vi "Get latest RSS.vi"(8 "error in (no error)":errorcluster, 10 "software sets":T1[](array[typedef]) {"information"."component type" items=["standard", "hidden", "system", "unknown", "startup"]; "items"."component type" items=["standard", "hidden", "system", "unknown", "startup"]; "add-ons"."component type" items=["standard", "hidden", "system", "unknown", "startup"]}) -> (0 "error out":errorcluster, 2 "software set":T1 {"information"."component type" items=["standard", "hidden", "system", "unknown", "startup"]; "items"."component type" items=["standard", "hidden", "system", "unknown", "startup"]; "add-ons"."component type" items=["standard", "hidden", "system", "unknown", "startup"]})   [LabVIEW 2016, in "RT Management.lvlib" / "RT Management.lvclass"]
uses:
  RT Management.lvclass
  <vilib>/nisyscfg/Software Set 1.2.ctl
  <vilib>/nisyscfg/Software 1.2.ctl
  <vilib>/nisyscfg/Component Type.ctl
  RT Management.lvlib
  <vilib>/nisyscfg/nisyscfg.lvlib
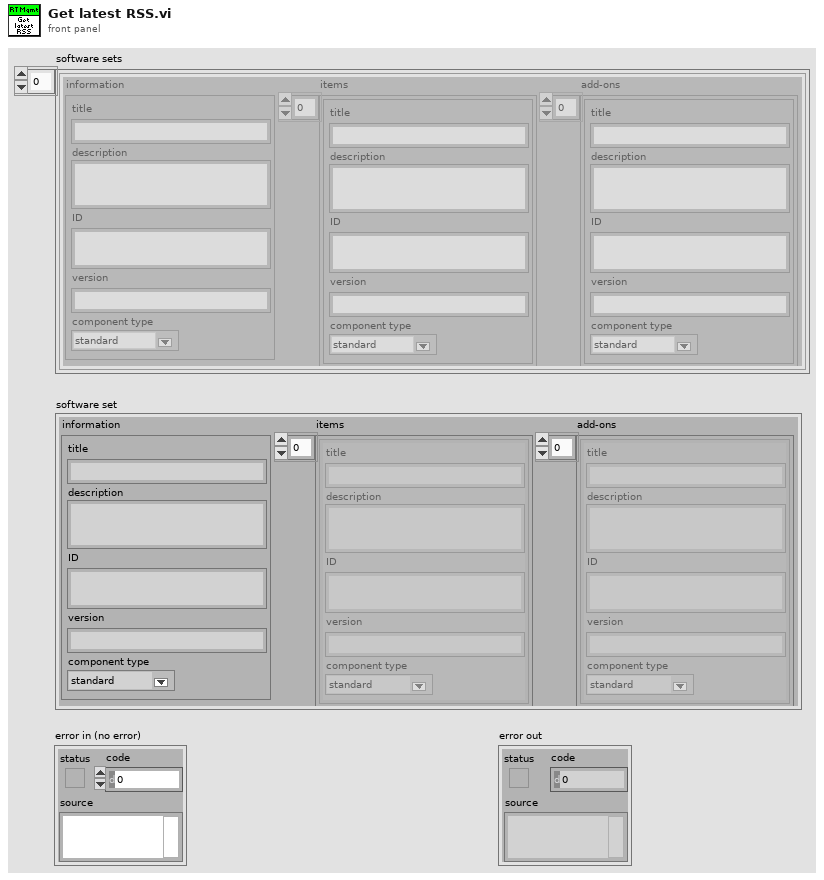
[diagram p1: front panel]
types:
  T1 = typedef "nisyscfg.lvlib/Software Set 1.2.ctl" = cluster{"information":T2, "items":T2[], "add-ons":T2[]}
  T2 = typedef "nisyscfg.lvlib/Software 1.2.ctl" = cluster{"title":string, "description":string, "ID":string, "version":string, "component type":T3}
  T3 = typedef "nisyscfg.lvlib/Component Type.ctl" = u32
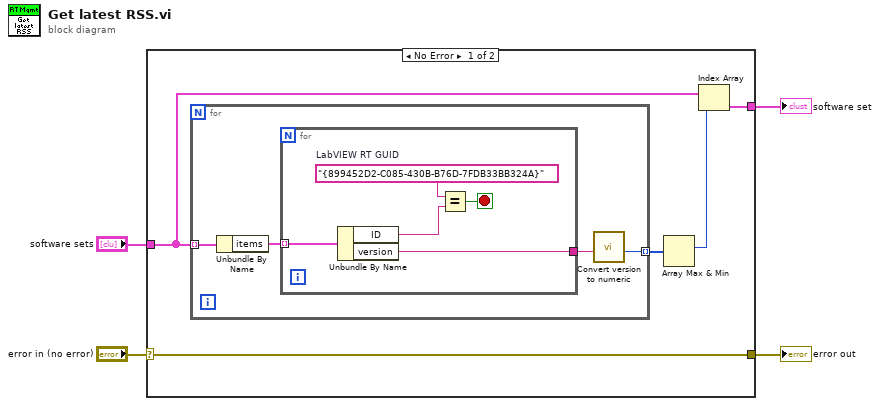
[diagram p0: block diagram]
diagram:
  n1 = case shown="No Error" "error in (no error)" {
    selector: "error in (no error)" -> [w9 w19]
    tunnel: [w9 w19] -> w3
    tunnel: "software sets" -> [w7 _]
    tunnel: [w5 _] -> w1
    frame No Error {
      n2 = for {
        tunnel: w7 -> [w11] mode=indexing
        tunnel: [w12] -> w8 mode=indexing
        n3 = Unbundle By Name(w11) -> ("items"=w10:T2[])
        n4 = for {
          tunnel: w10 -> [w18] mode=indexing
          tunnel: [w17] -> w13
          stop <- w14 stop-if-true
          w15 = "{899452D2-C085-430B-B76D-7FDB33BB324A}"  # LabVIEW RT GUID
          n5 = Unbundle By Name(w18) -> ("ID"=w16:string, "version"=w17:string)
          n6 = Equal?(x=w15, y=w16) -> (x = y?=w14:bool)
        }
        n7 = call "Convert version to numeric.vi"("Version-String"=w13) -> ("Version-Numeric"=w12:u32)  [unwired: 10 in]
      }
      n8 = Array Max & Min(array=w8) -> (max index (indices)=w6:i32)  [unwired: 3 out]
      n9 = Index Array(array=w7, index=w6) -> (element=w5:T1)
    }
    frame Error {
    }
  }
  "error out" <- w3
  "software set" <- w1
